vi "Reset.vi"(8 "error in (no error)":errorcluster, 11 "ThorlabsLabJack in":refnum<class "ThorlabsLabJack.lvclass">) -> (0 "error out":errorcluster, 3 "ThorlabsLabJack out":refnum<class "ThorlabsLabJack.lvclass">)   [LabVIEW 2018, in "ThorlabsLabJack.lvlib" / "ThorlabsLabJack.lvclass"]
uses:
  ThorlabsLabJack.lvclass
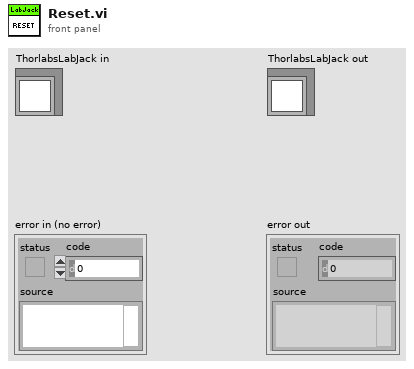
[diagram p1: front panel]
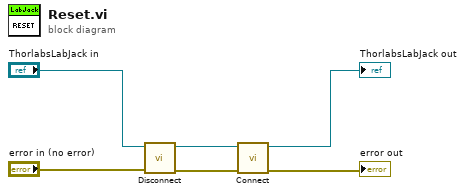
[diagram p0: block diagram]
diagram:
  n1 = call-dynamic "Disconnect.vi"("error in"="error in (no error)", "ThorlabsLabJack in"="ThorlabsLabJack in") -> ("error out"=w5:errorcluster, "ThorlabsLabJack out"=w1:refnum<class "ThorlabsLabJack.lvclass">)  [unwired: 8 in]
  n2 = call-dynamic "Connect.vi"("error in"=w5, "ThorlabsLabJack in"=w1) -> ("error out"=→"error out":errorcluster, "ThorlabsLabJack out"=→"ThorlabsLabJack out":refnum<class "ThorlabsLabJack.lvclass">)  [unwired: 8 in]
